vi "1.0 Testing Python Node VI.vi"() -> ()   [LabVIEW 2018]
panel:
  out "Array":dbl[](array[numeric])
  in  "module path":path
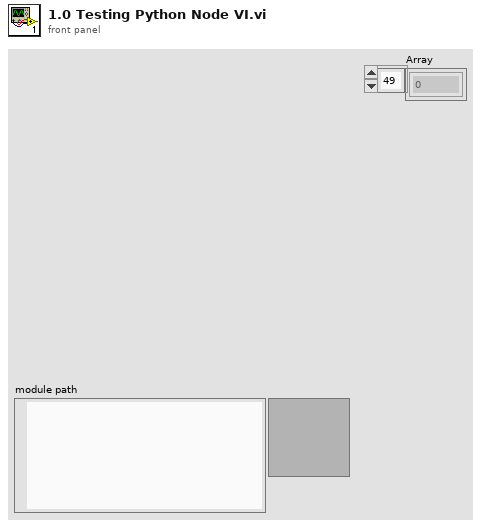
[diagram p1: front panel]
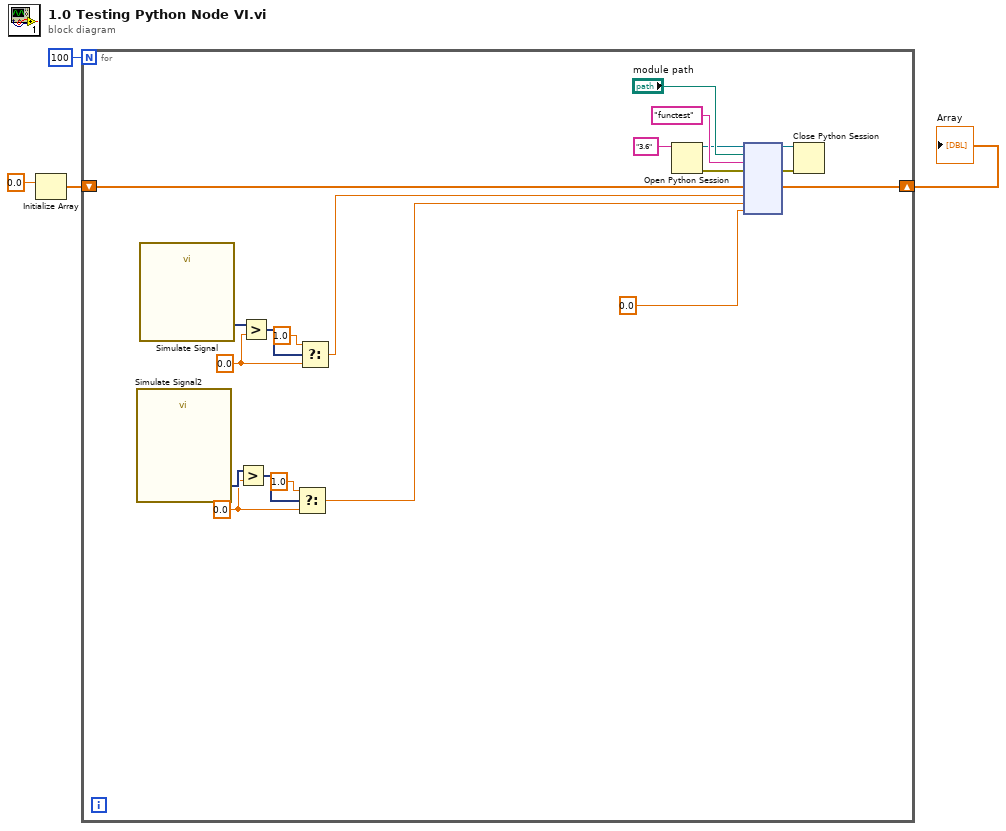
[diagram p0: block diagram]
diagram:
  n1 = Initialize Array(0.0) -> (w2:dbl[])  [unwired: 1 in]
  n2 = for {
    N: 100 -> [_]
    shift-right: [w12] -> w4
    shift-left: w2 -> [w13]
    w8 = 0.0 ("y")
    w21 = 0.0 ("y")
    n3 = call "Simulate Signal2"() -> ("Sine"=w11:dynamicdata)  [unwired: 14 in, 1 out]
    n4 = call "Simulate Signal"() -> ("Sine"=w24:dynamicdata)  [unwired: 14 in, 1 out]
    n5 = Greater?(x=w11, y=w8) -> (0:w10:dynamicdata)
    n6 = Greater?(x=w24, y=w21) -> (0:w23:dynamicdata)
    n7 = Select(t=1.0, s=w10, f=w8) -> (s? t:f=w7:dbl)
    n8 = Select(t=1.0, s=w23, f=w21) -> (s? t:f=w6:dbl)
    n9 = Open Python Session(python version="3.6" ("Python version")) -> (session out=w18:refnum<k35>, error out=w17:errorcluster)  [unwired: 2 in]
    n10 = node(w18, "module path", "functest" ("function name"), w17, w13, w6, w7, 0.0) -> (w15:refnum<k35>, w14:errorcluster, w12:dbl[])  [unwired: 5 in, 2 out]
    n11 = Close Python Session(session in=w15, error in=w14) -> ()  [unwired: 1 out]
  }
  "Array" <- w4
